vi "Part 1.vi"(11 "Input":string) -> (3 "Output":i64)   [LabVIEW 2021]
uses:
  <userlib>/_OpenG.lib/string/string.llb/Convert EOLs (String)__ogtk.vi
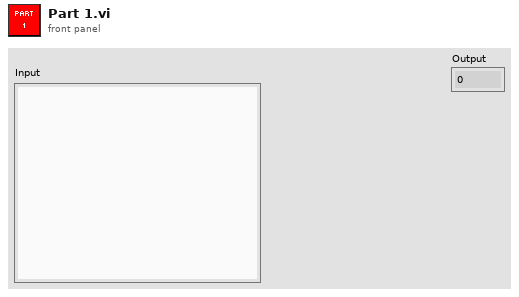
[diagram p1: front panel]
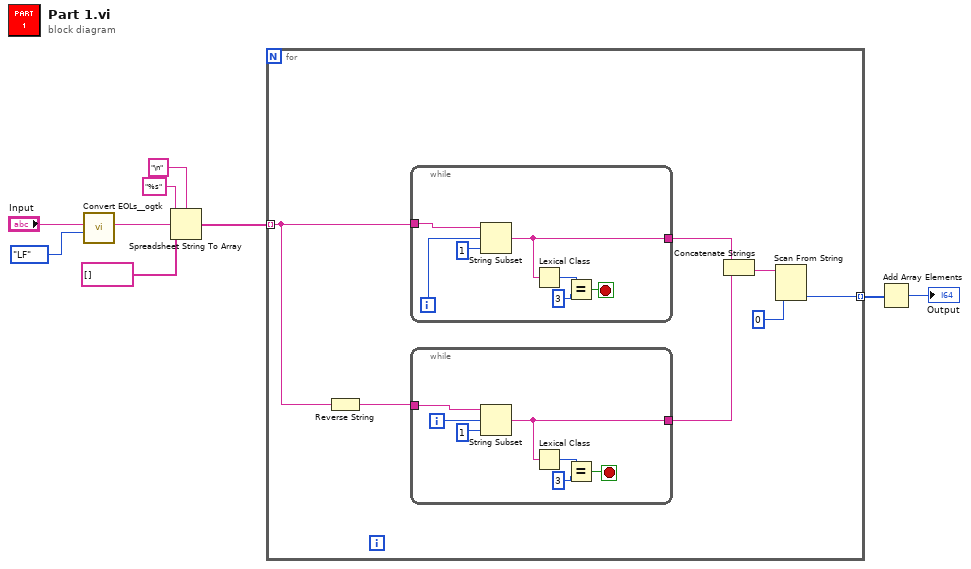
[diagram p0: block diagram]
diagram:
  n1 = call-poly <userlib>:"Convert EOLs__ogtk.vi"("Convert to:"=enum16{"CR", "LF", "CRLF"}."LF", "String in"="Input") -> ("String out"=w5:string)  [unwired: 9 in]
  n2 = Spreadsheet String To Array(delimiter (Tab)="\n", format string="%s", spreadsheet string=w5, array type (2D Dbl)=string[] []) -> (array=w3:string[])
  n3 = for {
    tunnel: w3 -> [w16] mode=indexing
    tunnel: [w14] -> w2 mode=indexing
    n4 = Reverse String(1:w16) -> (0:w12:string)
    n5 = while {
      tunnel: [w24] -> w11
      tunnel: w16 -> [w30]
      i -> [w28]
      stop <- w25 stop-if-true
      n6 = String Subset(string=w30, offset (0)=w28, length (rest)=1) -> (substring=w24:string)
      n7 = Lexical Class(1:w24) -> (0:w27:i16)
      n8 = Equal?(x=w27, y=3) -> (x = y?=w25:bool)
    }
    n9 = while {
      tunnel: [w17] -> w10
      tunnel: w12 -> [w23]
      i -> [w21]
      stop <- w18 stop-if-true
      n10 = String Subset(string=w23, offset (0)=w21, length (rest)=1) -> (substring=w17:string)
      n11 = Lexical Class(1:w17) -> (0:w20:i16)
      n12 = Equal?(x=w20, y=3) -> (x = y?=w18:bool)
    }
    n13 = Concatenate Strings(w11, w10) -> (w15:string)
    n14 = Scan From String(input string=w15, default 1=i64 0 ("Output")) -> (output 1=w14:i64)  [unwired: 3 in, 3 out]
  }
  n15 = Add Array Elements(numeric array=w2) -> (sum=→"Output":i64)
